vi "Connect.vi"(7 "command is subsystem":bool, 8 "error in (no error)":errorcluster, 9 "command":string, 10 "user@host":string, 11 "session in":refnum<class "Generic Client.lvclass">) -> (0 "error out":errorcluster, 2 "SSH subprocess":refnum<class "Subprocess.lvclass">, 3 "session out":refnum<class "Generic Client.lvclass">)   [LabVIEW 2020, in "NI_SSH.lvlib" / "Generic Client.lvclass"]
doc: "Connects to an SFTP server. The <b>client</b> determines which SSH Client to use."
uses:
  <vilib>/net/SSH/Client/Generic/Generic Client.lvclass
  <vilib>/Subprocess/Subprocess/Subprocess.lvclass
  <vilib>/net/SSH/Client/Generic/Generic Client.lvclass/Generic Client.ctl
  <vilib>/net/SSH/Client/Generic/Write user_host.vi
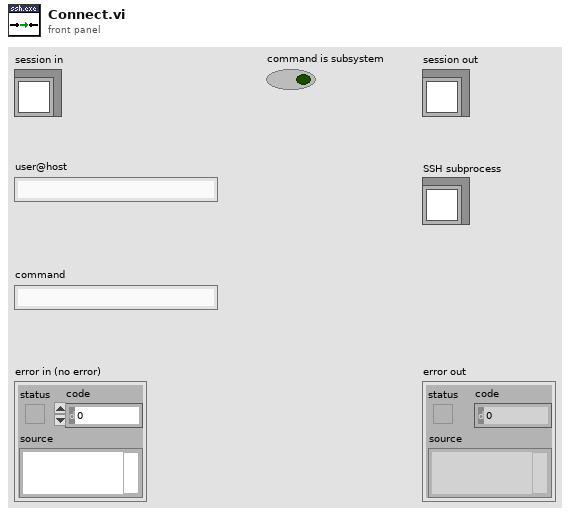
[diagram p1: front panel]
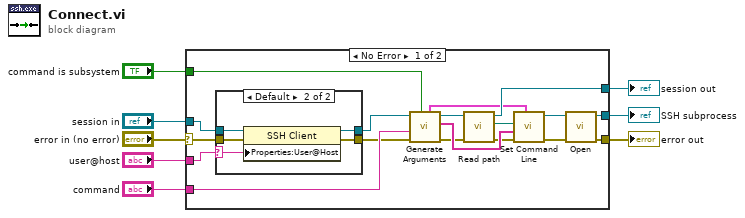
[diagram p0: block diagram]
diagram:
  n1 = case shown="No Error" "error in (no error)" {
    selector: "error in (no error)" -> [w11 w35]
    tunnel: [w22 w35] -> w8
    tunnel: [w21 _] -> w6
    tunnel: "session in" -> [w12 w34]
    tunnel: [w19 w34] -> w4
    tunnel: "user@host" -> [w9 _]
    tunnel: "command is subsystem" -> [w16 _]
    tunnel: "command" -> [w15 _]
    frame No Error {
      n2 = case shown="Default" w9 {
        selector: w9 -> [_ w29]
        tunnel: [w28 w33] -> w13
        tunnel: w12 -> [w28 w32]
        tunnel: w11 -> [w27 w31]
        tunnel: [w27 w30] -> w10
        frame "" {
        }
        frame Default {
          n3 = property class="SSH Client"(reference=w32, error in=w31, "Properties:User@Host"=w29) -> (reference out=w33:refnum<class "Generic Client.lvclass">, error out=w30:errorcluster)
        }
      }
      n4 = call-dynamic "Generate Arguments.vi"("subsystem?"=w16, "error in (no error)"=w10, "command"=w15, "client in"=w13) -> ("error out"=w18:errorcluster, "arguments"=w26:string[], "client out"=w20:refnum<class "Generic Client.lvclass">, "environment variables"=w14:cluster{"name":string, "value":string}[])  [unwired: 4 in]
      n5 = call-dynamic "Read path.vi"("error in (no error)"=w18, "Generic Client in"=w20) -> ("error out"=w17:errorcluster, "path"=w25:path, "Generic Client out"=w19:refnum<class "Generic Client.lvclass">)  [unwired: 7 in]
      n6 = call <vilib>:"Set Command Line.vi"("environment variables"=w14, "error in (no error)"=w17, "arguments"=w26, "path"=w25) -> ("error out"=w23:errorcluster, "subprocess out"=w24:refnum<class "Subprocess.lvclass">)  [unwired: 6 in]
      n7 = call <vilib>:"Open.vi"("error in (no error)"=w23, "subprocess in"=w24) -> ("error out"=w22:errorcluster, "subprocess out"=w21:refnum<class "Subprocess.lvclass">)  [unwired: 8 in]
    }
    frame Error {
    }
  }
  "error out" <- w8
  "session out" <- w4
  "SSH subprocess" <- w6
